vi "AMC Flush Message Queue.vi"(7 "error in (no error)":errorcluster, 10 "Message Queue in":T1) -> (0 "error out":errorcluster, 3 "Message Queue out":T1)   [LabVIEW 2017]
uses:
  subVIs/TypeDefs/amc_Message Queue.ctl
  subVIs/TypeDefs/amc_Message.ctl
  Tools/Keyed Array/Tools_KeyedArray KeyedArray.ctl
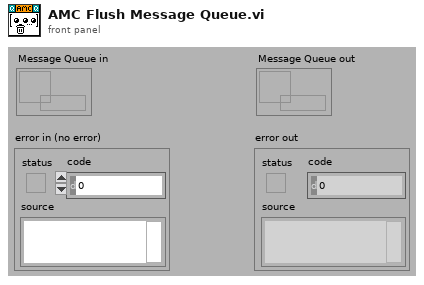
[diagram p1: front panel]
types:
  T1 = typedef "amc_Message Queue.ctl" = refnum<queue>
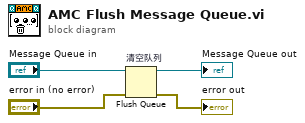
[diagram p0: block diagram]
diagram:
  n1 = Flush Queue "清空队列"(queue="Message Queue in", error in (no error)="error in (no error)") -> (queue out=→"Message Queue out":T1, error out=→"error out":errorcluster)  [unwired: 1 out]
